vi "CTR-Configure.vi"(7 "Sampling rate (Hz)":dbl, 9 "Npts":i32, 11 "error in (no error)":errorcluster) -> (15 "error out":errorcluster)   [LabVIEW 2020]
uses:
  Typedefs/CTR-Action.ctl
  Typedefs/CTR-Config.ctl
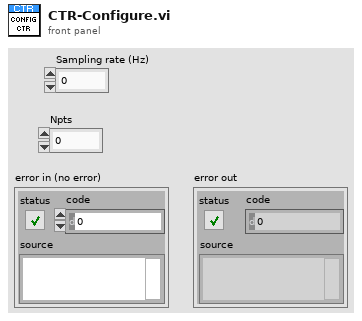
[diagram p1: front panel]
types:
  T1 = typedef "CTR-Action.ctl" = enum16{"Clear", "Configure", "Initialize", "Start", "Clean up"}
  T2 = typedef "CTR-Config.ctl" = cluster{"enabled":bool, "Hi ticks":u32, "Low ticks":u32, "Idle state":i32, "Delay ticks":u32}
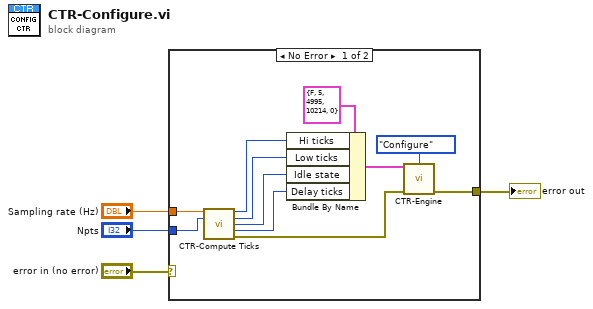
[diagram p0: block diagram]
diagram:
  n1 = case shown="No Error" "error in (no error)" {
    selector: "error in (no error)" -> [_ w16]
    tunnel: [w14 w16] -> w3
    tunnel: "Sampling rate (Hz)" -> [w11 _]
    tunnel: "Npts" -> [w10 _]
    frame No Error {
      n2 = call "CTR-Compute Ticks.vi"("Sampling Rate (Hz)"=w11, "Npts"=w10) -> ("Hi ticks"=w8:u32, "Low ticks"=w7:u32, "Idle state"=w6:i32, "Delay ticks"=w5:u32, "error out"=w9:errorcluster)  [unwired: 9 in]
      n3 = Bundle By Name(cluster=T2 {"enabled"=FALSE, "Hi ticks"=5, "Low ticks"=4995, "Idle state"=10214, "Delay ticks"=0} ("Config"), "Hi ticks"=w8, "Low ticks"=w7, "Idle state"=w6, "Delay ticks"=w5) -> (w12:T2)
      n4 = call "CTR-Engine.vi"("Config"=w12, "action"=CTR-Action."Configure", "error in (no error)"=w9) -> ("error out"=w14:errorcluster)  [unwired: 12 in]
    }
    frame Error {
    }
  }
  "error out" <- w3
